vi "更换刀具.vi"(8 "error in (no error)":errorcluster caption="错误输入（无错误）", 11 "加工中心 输入":refnum<class "加工中心.lvclass"> caption="DNL_LabVIEW Object in") -> (0 "error out":errorcluster caption="错误输出", 3 "加工中心 输出":refnum<class "加工中心.lvclass"> caption="DNL_LabVIEW Object out")   [LabVIEW 2011, in "加工中心.lvclass"]
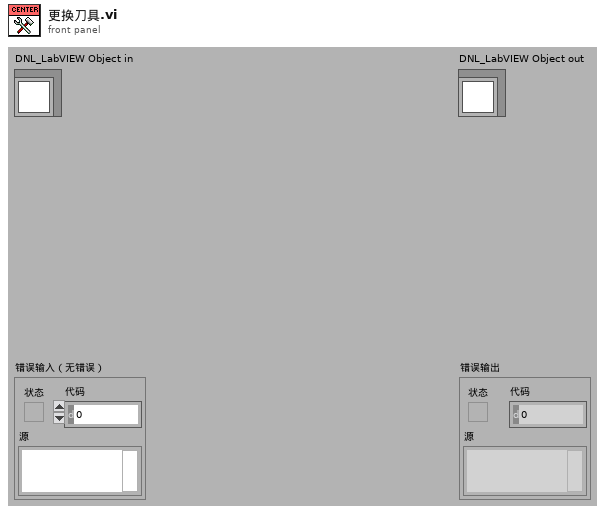
[diagram p1: front panel]
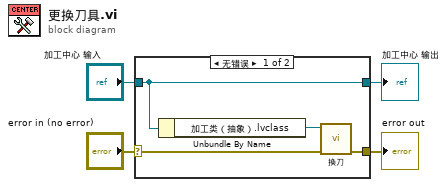
[diagram p0: block diagram]
diagram:
  n1 = case shown="无错误" "error in (no error)" {
    selector: "error in (no error)" -> [w6 w10]
    tunnel: [w5 w10] -> w3
    tunnel: [w8 w9] -> w1
    tunnel: "加工中心 输入" -> [w8 w9]
    frame No Error {
      n2 = Unbundle By Name(w8) -> ("加工类（抽象）.lvclass"=w7:refnum<class "加工类（抽象）.lvclass">)
      n3 = call-dynamic "换刀.vi"("error in (no error)"=w6, "加工类（抽象） 输入"=w7) -> ("error out"=w5:errorcluster)  [unwired: 8 in, 1 out]
    }
    frame Error {
    }
  }
  "error out" <- w3
  "加工中心 输出" <- w1
